vi "calculate cross correlation.vi"(8 "error in (no error)":errorcluster, 11 "Thorcam in":refnum<class "Thorcam.lvclass">) -> (0 "error out":errorcluster, 3 "Thorcam out":refnum<class "Thorcam.lvclass">)   [LabVIEW 2012, in "Thorcam.lvclass"]
uses:
  Thorcam.lvclass
  Thorcam.lvclass/Thorcam.ctl
  <vilib>/vision/NI_Vision_Development_Module.lvlib
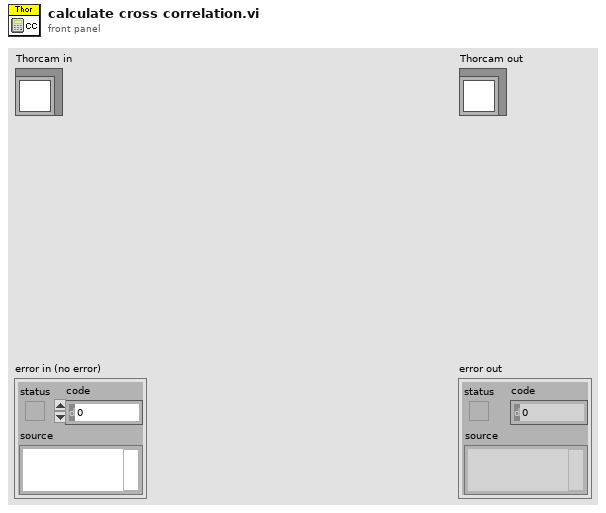
[diagram p1: front panel]
types:
  T1 = cluster{"Sampling Percentage":dbl, "maximum iteration":i32, "number of bins":u32}
  T2 = typedef "Thorcam.lvclass/cross correlation method.ctl" = enum16{"default", "normalised cross correlation", "normalised mutual information"}
  T3 = typedef "IMAQ Image.ctl" = refnum<image>
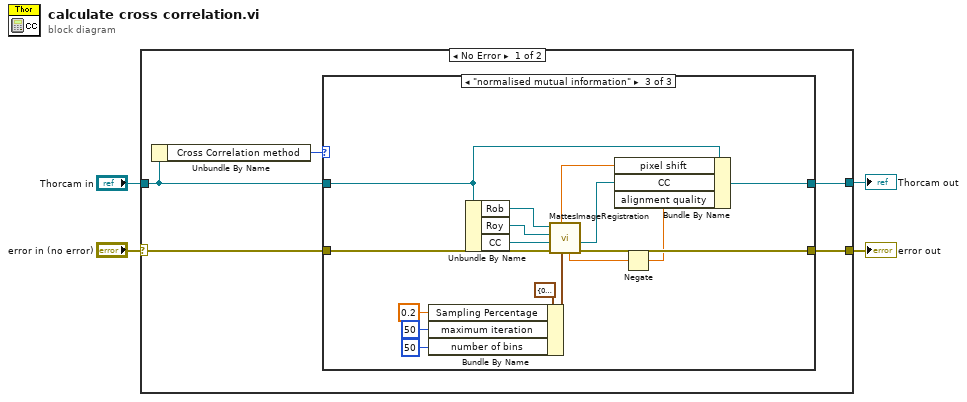
[diagram p0: block diagram]
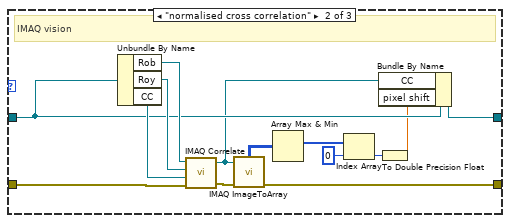
[diagram p3: hidden frame]
diagram:
  n1 = case shown="No Error" "error in (no error)" {
    selector: "error in (no error)" -> [w5 w43]
    tunnel: [w7 w43] -> w3
    tunnel: [w8 w42] -> w1
    tunnel: "Thorcam in" -> [w6 w42]
    frame No Error {
      n2 = Unbundle By Name(w6) -> ("Cross Correlation method"=w9:T2)
      n3 = case shown="\"normalised mutual information\"" w9 {
        tunnel: w6 -> [w11 w16 w37]
        tunnel: [w11 w15 w36] -> w8
        tunnel: w5 -> [w10 w25 w41]
        tunnel: [w10 w13 w38] -> w7
        frame "default", Default {
        }
        frame "normalised cross correlation" {
          # "IMAQ vision"
          n4 = Unbundle By Name(w16) -> ("Rob"=w24:T3, "Roy"=w23:T3, "CC"=w22:T3)
          n5 = call "IMAQ Correlate"("Image Src"=w24, "Image Template"=w23, "Image Dst"=w22, "error in (no error)"=w25) -> ("Image Dst Out"=w12:T3, "error out"=w21:errorcluster)  [unwired: 3 in]
          n6 = call "IMAQ ImageToArray"("error in (no error)"=w21, "Image"=w12) -> ("error out"=w13:errorcluster, "Image Pixels (U8)"=w20:u8[][])  [unwired: 2 in, 3 out]
          n7 = Array Max & Min(array=w20) -> (max index (indices)=w19:i32[])  [unwired: 3 out]
          n8 = Index Array(array=w19, index=0) -> (element=w17:i32)
          n9 = To Double Precision Float(number=w17) -> (double precision float=w14:dbl)
          n10 = Bundle By Name(cluster=w16, "CC"=w12, "pixel shift"=w14) -> (w15:refnum<class "Thorcam.lvclass">)
        }
        frame "normalised mutual information" {
          n11 = Bundle By Name(cluster=T1 {"Sampling Percentage"=0.2, "maximum iteration"=200, "number of bins"=200} ("Registration parameters"), "Sampling Percentage"=0.2, "maximum iteration"=50, "number of bins"=u32 50) -> (w30:T1)
          n12 = Unbundle By Name(w37) -> ("Rob"=w40:T3, "Roy"=w39:T3, "CC"=w32:T3)
          n13 = call "MattesImageRegistration.vi"("Registration parameters"=w30, "error in (no error)"=w41, "False color image in"=w32, "Moving image in"=w39, "Fixed image in"=w40) -> ("error out"=w38:errorcluster, "False color alignment image"=w35:T3, "alignment quality"=w33:dbl, "x translation"=w34:dbl)  [unwired: 3 out]
          n14 = Negate(x=w33) -> (-x=w26:dbl)
          n15 = Bundle By Name(cluster=w37, "pixel shift"=w34, "CC"=w35, "alignment quality"=w26) -> (w36:refnum<class "Thorcam.lvclass">)
        }
      }
    }
    frame Error {
    }
  }
  "error out" <- w3
  "Thorcam out" <- w1
